vi "_GetCalFiles.vi"(7 "CalOption":enum32{"Positive", "Negative"}(radio)) -> (0 "error out":errorcluster, 1 "SystemInfo":string, 2 "oldTablePath":path, 3 "calFiles":path[](array[path]), 4 "OtherDirectories":path[](array[path]), 5 "Model Name":T1=enum."IONICS 3Q 210")   [LabVIEW 2015]
uses:
  Type/_Instrument Model.ctl
  Type/_Log Command.ctl
  Type/_SaveOption.ctl
  Configuration/_Global Configuration.vi
  <vilib>/Utility/config.llb/Read Key (Path).vi
  <vilib>/Utility/config.llb/NI_LVConfig.lvlib
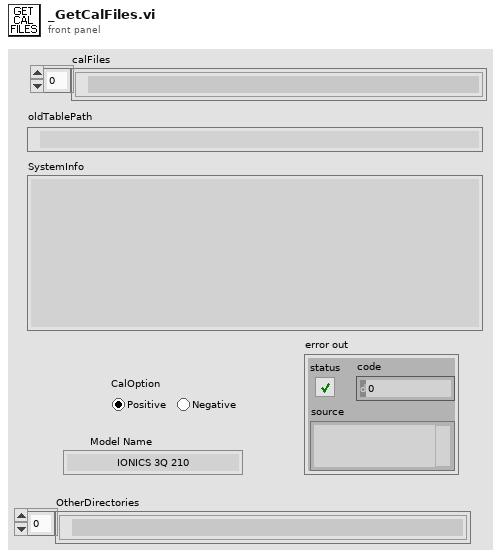
[diagram p1: front panel]
types:
  T1 = typedef "_Instrument Model.ctl" = enum16{"QSight 110", "QSight 120", "QSight 210", "QSight 220", "IONICS 3Q 110", "IONICS 3Q 120", "IONICS 3Q 210", "IONICS 3Q 220", "IONICS 3Q 310", "IONICS 3Q 320", "Simulation (Single Source)", "Simulation (Dual Source)"}
  T2 = typedef "_Log Command.ctl" = enum16{"No Command", "Open", "Read", "Write", "Close", "Check Size"}
  T3 = typedef "NI_LVConfig.lvlib/Config Data RefNum.ctl" = refnum<k1>
  T4 = typedef "_RT Instrument 2.ctl" = cluster{"Table":T5[], "Instrument":string[]}
  T5 = typedef "_RT Configuration 2.ctl" = cluster{"Name":string, "Ch#":u8, "Min":dbl, "Max":dbl, "Def+":dbl, "Def-":dbl, "Offset":dbl, "Slope":dbl, "Type":u8, "Description":string, "SettleT":dbl}
  T6 = typedef "_SaveOption.ctl" = enum16{"Use Dialog", "Temporary File", "My Tables", "Full Path"}
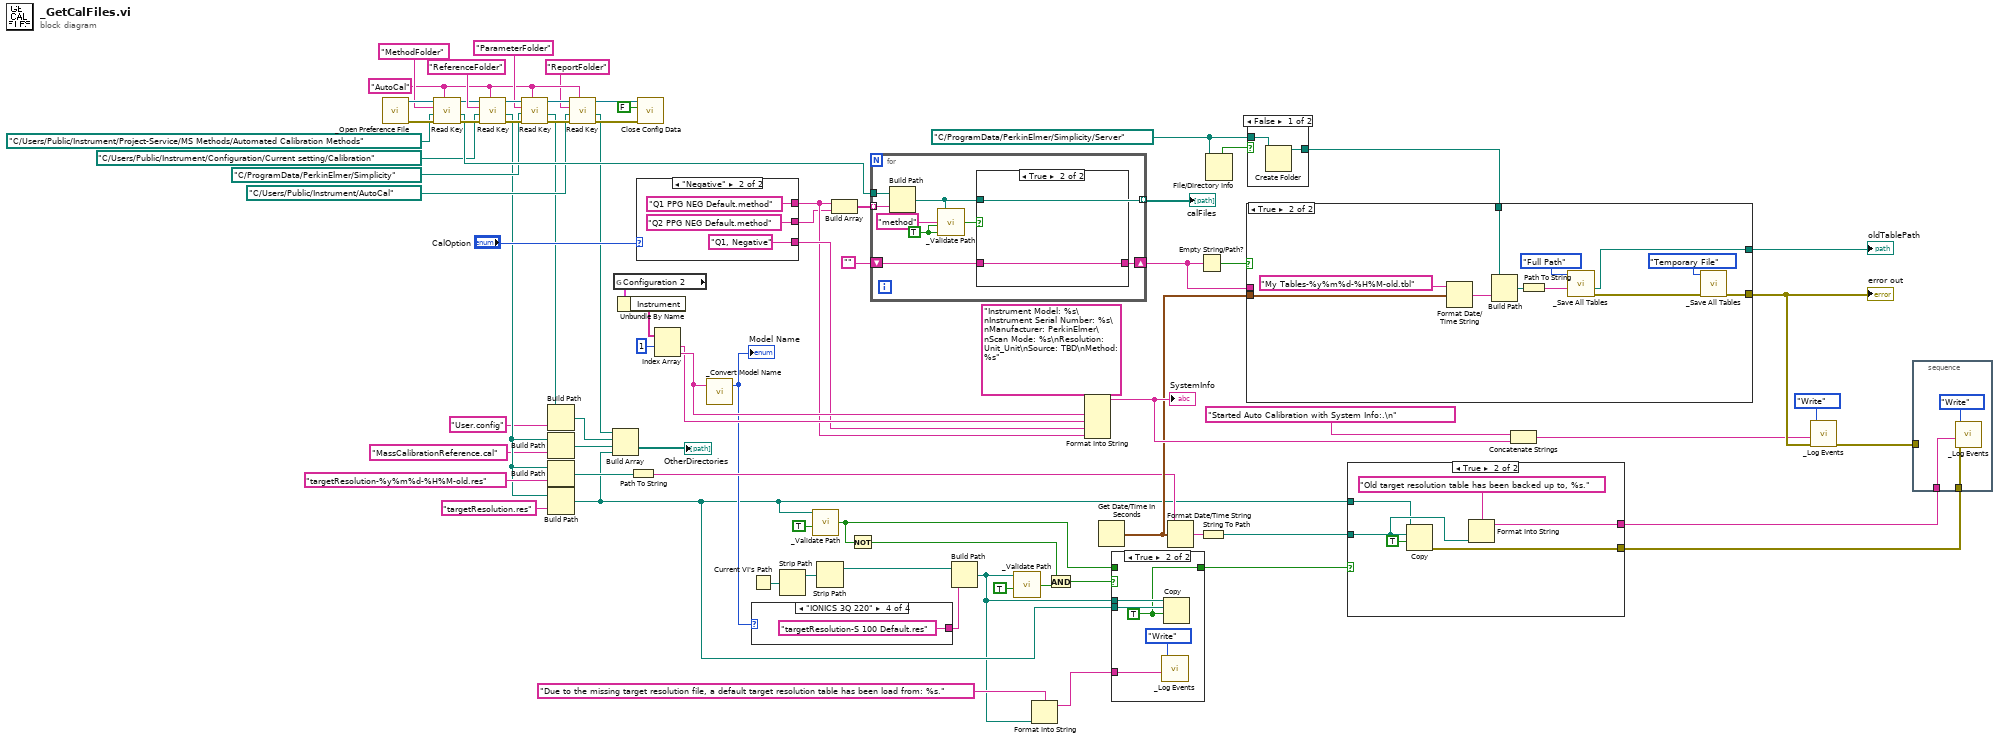
[diagram p0: block diagram]
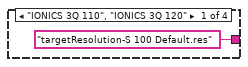
[diagram p3: hidden frame]
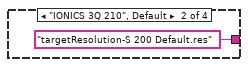
[diagram p4: hidden frame]
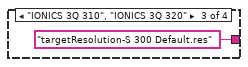
[diagram p5: hidden frame]
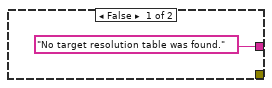
[diagram p6: hidden frame]
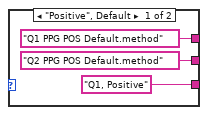
[diagram p8: hidden frame]
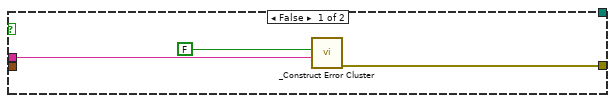
[diagram p9: hidden frame]
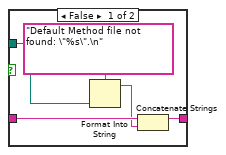
[diagram p10: hidden frame]
diagram:
  w17 = path "C:/ProgramData/PerkinElmer/Simplicity/Server" ("appended path")
  w38 = "AutoCal" ("section")
  n1 = call "_Open Preference File.vi"() -> ("error"=w46:errorcluster, "refnum"=w50:T3)  [unwired: 3 in, 3 out]
  n2 = call-poly <vilib>:"Read Key.vi"("section"=w38, "error in (no error)"=w46, "default value"=path "C:/Users/Public/Instrument/Project-Service/MS Methods/Automated Calibration Methods" ("oldTablePath"), "key"="MethodFolder" ("section"), "refnum"=w50) -> ("error out"=w45:errorcluster, "value"=w33:path, "refnum out"=w47:T3)  [unwired: 3 in, 1 out]
  n3 = call-poly <vilib>:"Read Key.vi"("section"=w38, "error in (no error)"=w45, "default value"=path "C:/Users/Public/Instrument/Configuration/Current setting/Calibration" ("path"), "key"="ReferenceFolder" ("section"), "refnum"=w47) -> ("error out"=w43:errorcluster, "value"=w25:path, "refnum out"=w42:T3)  [unwired: 3 in, 1 out]
  n4 = call-poly <vilib>:"Read Key.vi"("section"=w38, "error in (no error)"=w43, "default value"=path "C:/ProgramData/PerkinElmer/Simplicity" ("path"), "key"="ParameterFolder" ("section"), "refnum"=w42) -> ("error out"=w40:errorcluster, "value"=w22:path, "refnum out"=w39:T3)  [unwired: 3 in, 1 out]
  n5 = Build Path(base path=w22, name or relative path="User.config" ("time format string (%c)")) -> (appended path=w20:path)
  n6 = Build Path(base path=w25, name or relative path="MassCalibrationReference.cal" ("time format string (%c)")) -> (appended path=w21:path)
  n7 = Build Path(base path=w25, name or relative path="targetResolution-%y%m%d-%H%M-old.res" ("time format string (%c)")) -> (appended path=w28:path)
  n8 = Build Path(base path=w25, name or relative path="targetResolution.res" ("time format string (%c)")) -> (appended path=w8:path)
  n9 = call-poly <vilib>:"Read Key.vi"("section"=w38, "error in (no error)"=w40, "default value"=path "C:/Users/Public/Instrument/AutoCal" ("path"), "key"="ReportFolder" ("section"), "refnum"=w39) -> ("error out"=w35:errorcluster, "value"=w19:path, "refnum out"=w36:T3)  [unwired: 3 in, 1 out]
  n10 = Build Array(w19, w20, w21, w8) -> (→"OtherDirectories":path[])
  n11 = global read "_Global Configuration.vi" "Configuration 2"() -> (w79:T4)
  n12 = Unbundle By Name(w79) -> ("Instrument"=w78:string[])
  n13 = Path To String(path=w28) -> (string=w27:string)
  n14 = case shown="\"Negative\"" "CalOption" {
    tunnel: ["Q1 PPG POS Default.method" ("time format string (%c)") "Q1 PPG NEG Default.method" ("time format string (%c)")] -> w65
    tunnel: ["Q2 PPG POS Default.method" ("time format string (%c)") "Q2 PPG NEG Default.method" ("time format string (%c)")] -> w64
    tunnel: ["Q1, Positive" ("time format string (%c)") "Q1, Negative" ("time format string (%c)")] -> w68
    frame "Positive", Default {
    }
    frame "Negative" {
    }
  }
  n15 = call <vilib>:"Close Config Data.vi"("error in (no error)"=w35, "write file if changed (T)"=FALSE, "refnum"=w36) -> ()  [unwired: 9 out]
  n16 = Index Array(array=w78, index #1=1 ("index")) -> (element #1=w69:string, element #2=w70:string)  [unwired: 1 in]
  n17 = call "_Convert Model Name.vi"("Model"=w70) -> ("Model Name"=w16:T1)  [unwired: 1 in, 1 out]
  "Model Name" <- w16
  n18 = Current VI's Path() -> (path=w15:path)
  n19 = case shown="\"IONICS 3Q 220\"" w16 {
    tunnel: ["targetResolution-S 100 Default.res" ("time format string (%c)") "targetResolution-S 200 Default.res" ("time format string (%c)") "targetResolution-S 300 Default.res" ("time format string (%c)") "targetResolution-S 100 Default.res" ("time format string (%c)")] -> w12
    frame "IONICS 3Q 110", "IONICS 3Q 120" {
    }
    frame "IONICS 3Q 210", Default {
    }
    frame "IONICS 3Q 310", "IONICS 3Q 320" {
    }
    frame "IONICS 3Q 220" {
    }
  }
  n20 = Strip Path(path=w15) -> (stripped path=w14:path)  [unwired: 1 out]
  n21 = call "_Validate Path.vi"("Check Exist (F)"=TRUE, "path"=w8) -> ("Valid"=w5:bool)  [unwired: 2 in]
  n22 = Strip Path(path=w14) -> (stripped path=w13:path)  [unwired: 1 out]
  n23 = Build Array(w65, w64) -> (w76:string[])
  n24 = Not(x=w5) -> (.not. x?=w7:bool)
  n25 = for {
    tunnel: w76 -> [w97] mode=indexing
    tunnel: w33 -> [w96]
    tunnel: [w92] -> w63 mode=indexing
    shift-right: [w90] -> w73
    shift-left: "" -> [w91]
    w94 = TRUE ("Check Type (F)")
    n26 = Build Path(base path=w96, name or relative path=w97) -> (appended path=w92:path)
    n27 = call "_Validate Path.vi"("Check Type (F)"=w94, "Check Exist (F)"=w94, "Type (isd)"="method", "path"=w92) -> ("Valid"=w93:bool)
    n28 = case shown="True" w93 {
      tunnel: w92 -> [w102 _]
      tunnel: w91 -> [w100 w103]
      tunnel: [w98 w103] -> w90
      frame False {
        n29 = Format Into String(format string="Default Method file not found: \"%s\".\n", w102) -> (resulting string=w99:string)  [unwired: 2 in, 1 out]
        n30 = Concatenate Strings(w100, w99) -> (w98:string)
      }
      frame True {
      }
    }
  }
  "calFiles" <- w63
  n31 = Build Path(base path=w13, name or relative path=w12) -> (appended path=w3:path)
  n32 = call "_Validate Path.vi"("Check Exist (F)"=TRUE, "path"=w3) -> ("Valid"=w10:bool)  [unwired: 2 in]
  n33 = Format Into String(format string="Due to the missing target resolution file, a default target resolution table has been load from: %s." ("initial string"), w3) -> (resulting string=w2:string)  [unwired: 2 in, 1 out]
  n34 = And(x=w7, y=w10) -> (x .and. y?=w9:bool)
  n35 = Format Into String(format string="Instrument Model: %s\nInstrument Serial Number: %s\nManufacturer: PerkinElmer\nScan Mode: %s\nResolution: Unit_Unit\nSource: TBD\nMethod: %s" ("SystemInfo"), w70, w69, w68, w65) -> (resulting string=w59:string)  [unwired: 2 in, 1 out]
  "SystemInfo" <- w59
  n36 = Get Date/Time In Seconds() -> (seconds since 1Jan1904=w57:timestamp)
  n37 = case shown="True" w9 {
    tunnel: w3 -> [_ w109]
    tunnel: w8 -> [_ w108]
    tunnel: [w104 w107] -> w6
    tunnel: w5 -> [w104 _]
    tunnel: w2 -> [_ w105]
    frame False {
    }
    frame True {
      w107 = TRUE ("overwrite (F)")
      n38 = call "_Log Events.vi"("Event"=w105, "Log Command"=_Log_Command."Write" ("File Command")) -> ()  [unwired: 6 in, 2 out]
      n39 = Copy(9:w107, 10:w108, 11:w109) -> ()  [unwired: 1 in, 4 out]
    }
  }
  n40 = Format Date/Time String(time format string (%c)=w27, seconds (now)=w57) -> (date/time string=w56:string)  [unwired: 1 in]
  n41 = Empty String/Path?(string/path=w73) -> (empty?=w74:bool)
  n42 = String To Path(string=w56) -> (path=w53:path)
  n43 = File/Directory Info(path=w17) -> (directory=w67:bool)  [unwired: 1 in, 6 out]
  n44 = case shown="False" w67 {
    tunnel: w17 -> [w111 w112]
    tunnel: [w110 w112] -> w66
    frame False {
      n45 = Create Folder(path (use dialog)=w111) -> (created path=w110:path)  [unwired: 2 in, 2 out]
    }
    frame True {
    }
  }
  n46 = case shown="True" w74 {
    tunnel: w73 -> [w113 _]
    tunnel: [w115 w124] -> w61
    tunnel: w66 -> [_ w121]
    tunnel: w57 -> [_ w117]
    tunnel: [_ w116] -> w1
    frame False {
      n47 = call "_Construct Error Cluster.vi"("reason"=w113, "CallingChain? (T)"=FALSE) -> ("error out"=w115:errorcluster)  [unwired: 5 in]
    }
    frame True {
      n48 = Format Date/Time String(time format string (%c)="My Tables-%y%m%d-%H%M-old.tbl", seconds (now)=w117) -> (date/time string=w120:string)  [unwired: 1 in]
      n49 = Build Path(base path=w121, name or relative path=w120) -> (appended path=w119:path)
      n50 = Path To String(path=w119) -> (string=w118:string)
      n51 = call "_Save All Tables.vi"("FilePath(My Table.tbl)"=w118, "SaveOption (Temporary File)"=_SaveOption."Full Path" ("Use temporary file (F)")) -> ("error out"=w123:errorcluster, "Path"=w116:path)  [unwired: 1 in, 3 out]
      n52 = call "_Save All Tables.vi"("error in (no error)"=w123, "SaveOption (Temporary File)"=_SaveOption."Temporary File" ("Use temporary file (F)")) -> ("error out"=w124:errorcluster)  [unwired: 1 in, 4 out]
    }
  }
  "error out" <- w61
  "oldTablePath" <- w1
  n53 = case shown="True" w6 {
    tunnel: [_ w132] -> w54
    tunnel: w53 -> [_ w130]
    tunnel: ["No target resolution table was found." ("initial string") w129] -> w52
    tunnel: w8 -> [_ w128]
    frame False {
    }
    frame True {
      n54 = Copy(9:TRUE ("overwrite (F)"), 10:w130, 11:w128) -> (0:w132:errorcluster)  [unwired: 1 in, 3 out]
      n55 = Format Into String(format string="Old target resolution table has been backed up to, %s." ("initial string"), w130) -> (resulting string=w129:string)  [unwired: 2 in, 1 out]
    }
  }
  n56 = Concatenate Strings("Started Auto Calibration with System Info:.\n" ("format string"), w59) -> (w58:string)
  n57 = call "_Log Events.vi"("error in (no error)"=w61, "Event"=w58, "Log Command"=_Log_Command."Write" ("File Command")) -> ("error out"=w55:errorcluster)  [unwired: 5 in, 1 out]
  n58 = stacked-sequence {
    tunnel: w54 -> [w135]
    tunnel: w55 -> [_]
    tunnel: w52 -> [w134]
    frame #0 {
      n59 = call "_Log Events.vi"("error in (no error)"=w135, "Event"=w134, "Log Command"=_Log_Command."Write" ("File Command")) -> ()  [unwired: 5 in, 2 out]
    }
  }
